vi "ApplyLayoutToObject.vi"(5 "scaling settings":T1={"scaling factor"={"horizontal"=1.0, "vertical"=1.0}, "scaling to ignore"=variant} {"scaling factor"."vertical" min=0.0; "scaling factor"."horizontal" min=0.0}, 7 "properties to ignore":variant, 8 "error in (no error)":errorcluster, 10 "GObj Refnum":refnum<vi>, 11 "Array Control Layout in":refnum<class "Array Control Layout.lvclass">) -> (0 "error out":errorcluster, 3 "Array Control Layout out":refnum<class "Array Control Layout.lvclass">)   [LabVIEW 2010, in "NI_SE_Front Panel Layout.lvlib" / "Array Control Layout.lvclass"]
doc: "Apply layout information to the GObj Refnum."
uses:
  Array Control Layout.lvclass
  Scaling Factor_Options.ctl
  XY Scaling Factor.ctl
  Control Layout/Control Layout.lvclass
  Array Control Layout.lvclass/Array Control Layout.ctl
  Object Layout/Object Layout.lvclass
  Properties To Ignore.vi
  NI_SE_Front Panel Layout.lvlib
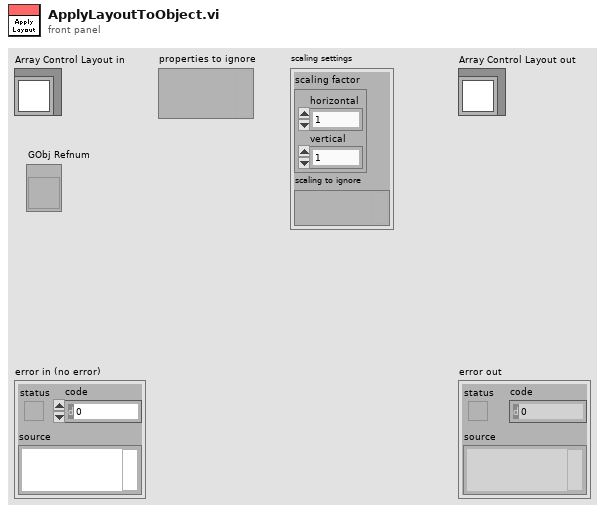
[diagram p1: front panel]
types:
  T1 = typedef "NI_SE_Front Panel Layout.lvlib/Scaling Factor_Options.ctl" = cluster{"scaling factor":T2, "scaling to ignore":variant}
  T2 = typedef "NI_SE_Front Panel Layout.lvlib/XY Scaling Factor.ctl" = cluster{"horizontal":dbl, "vertical":dbl}
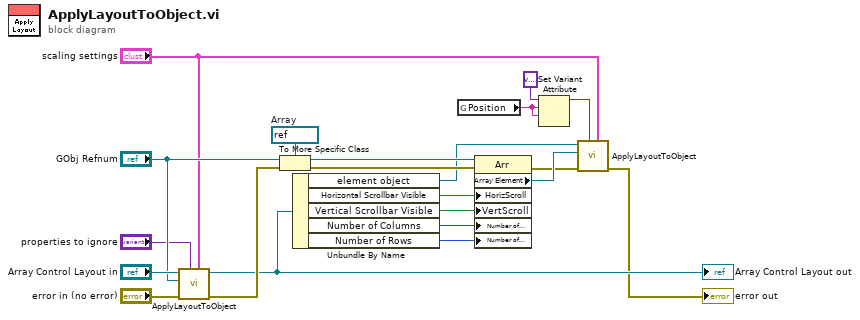
[diagram p0: block diagram]
diagram:
  w13 = refnum<vi> refnum  # Array
  n1 = call-parent "ApplyLayoutToObject.vi"("scaling settings"="scaling settings", "properties to ignore"="properties to ignore", "error in (no error)"="error in (no error)", "GObj Refnum"="GObj Refnum", "Control Layout in"="Array Control Layout in") -> ("error out"=w19:errorcluster, "Control Layout out"=w18:refnum<class "Array Control Layout.lvclass">)  [unwired: 5 in]
  "Array Control Layout out" <- w18
  n2 = To More Specific Class(target class=w13, reference="GObj Refnum", error in=w19) -> (specific class reference=w12:refnum<vi>, error out=w11:errorcluster)
  n3 = Unbundle By Name(w18) -> ("element object"=w10:refnum<class "Object Layout.lvclass">, "Horizontal Scrollbar Visible"=w5:bool, "Vertical Scrollbar Visible"=w4:bool, "Number of Columns"=w3:u32, "Number of Rows"=w2:u32)
  n4 = global read "Properties To Ignore.vi" "Position"() -> (w1:string)
  n5 = property class="Arr"(reference=w12, error in=w11, "HorizScroll"=w5, "VertScroll"=w4, "Number of Columns"=w3, "Number of Rows"=w2) -> (error out=w8:errorcluster, "Array Element"=w9:refnum<vi>)  [unwired: 1 out]
  n6 = Set Variant Attribute(Variant=variant ("properties to ignore"), name=w1, value=w1) -> (Variant out=w6:variant)  [unwired: 1 in, 2 out]
  n7 = call-dynamic "ApplyLayoutToObject.vi"("scaling settings"="scaling settings", "properties to ignore"=w6, "error in (no error)"=w8, "GObj Refnum"=w9, "Object Layout in"=w10) -> ("error out"=→"error out":errorcluster)  [unwired: 5 in, 1 out]
